vi "Interface.vi"() -> ()   [LabVIEW 2019]
uses:
  <vilib>/Instr/_visa.llb/VISA Configure Serial Port (Instr).vi
  <vilib>/addons/database/Connection.llb/DB Tools Open Connec (Path).vi
  <vilib>/addons/database/Connection.llb/Conn Execute.vi
  <vilib>/addons/database/Recordset.llb/Rec Destroy - Connection.vi
  <vilib>/addons/database/NI_Database_API.lvlib
panel:
  in  "stop":bool
  in  "Pagina":i16(slide) scale=1.0..3.0
  in  "Tab Control":enum32{"INTERFAZ", "ESQUEMA", "INSTRUCCIONES"}(tab)
  in  "VISA resource name":refnum<visa-resource-name>="COM5"
  out "Rt":dbl=100.0 format="%#.2g"
  out "Lectura":dbl
  out "T":dbl=-3.0 format="%#_4g"
  out "Waveform Chart":dbl(graph)=-3.0
  out "Termometro":dbl(slide)=-3.0 scale=10.0..60.0
  # "1.-INTERFAZ\n2.-ESQUEMA\n3.-INSTRUCCIONES"
  # "PÁGINA"
  # "VALORES"
  # "INTERFAZ"
  # "V"
  # "Instrucciones de\nUso en la página 3"
  # "VOLTAJE VAB"
  # "Ohm"
  # "RESISTENCIA PT100"
  # "ºC"
  # "TEMPERATURA"
  # "CIFPN1 Santander"
  # "CONFIGURACIÓN"
  # "(C) 2019"
  # "PUERTO SERIE"
  # "ALBANO DÍEZ DE PAULINO"
  # "ESQUEMA"
  # "Montar como se indica para que funcione correctamente"
  # "Adaptador DB9-USB"
  # "D"
  # "CIFPN1 Santander"
  # "uC ATMEGA328P"
  # "PT100"
  # "C"
  # "5V"
  # "Adaptador TTL-RS232/DB9"
  # "PC"
  # "Puente de Wilson"
  # "D"
  # "C"
  # "INSTRUCCIONES"
  # "Pasos previos antes de ejecutar VI"
  # "INSTRUCCIONES"
  # "1.-Borrar todas las tablas de la base de datos"
  # "1.-Ejecutar VI"
  # "2.-Seleccionar Puerto COM"
  # "2.-No tocar el control del Puerto Serie"
  # "3.-Observar los datos en la grafica y en el termometro"
  # "4.-(Opcional) Parar el programa con el boton STOP"
  # "5.-Esperar a que finalice el programa pasados 5 minutos"
  # "CIFPN1 Santander"
  # "(C) 2019"
  # "ALBANO DÍEZ DE PAULINO"
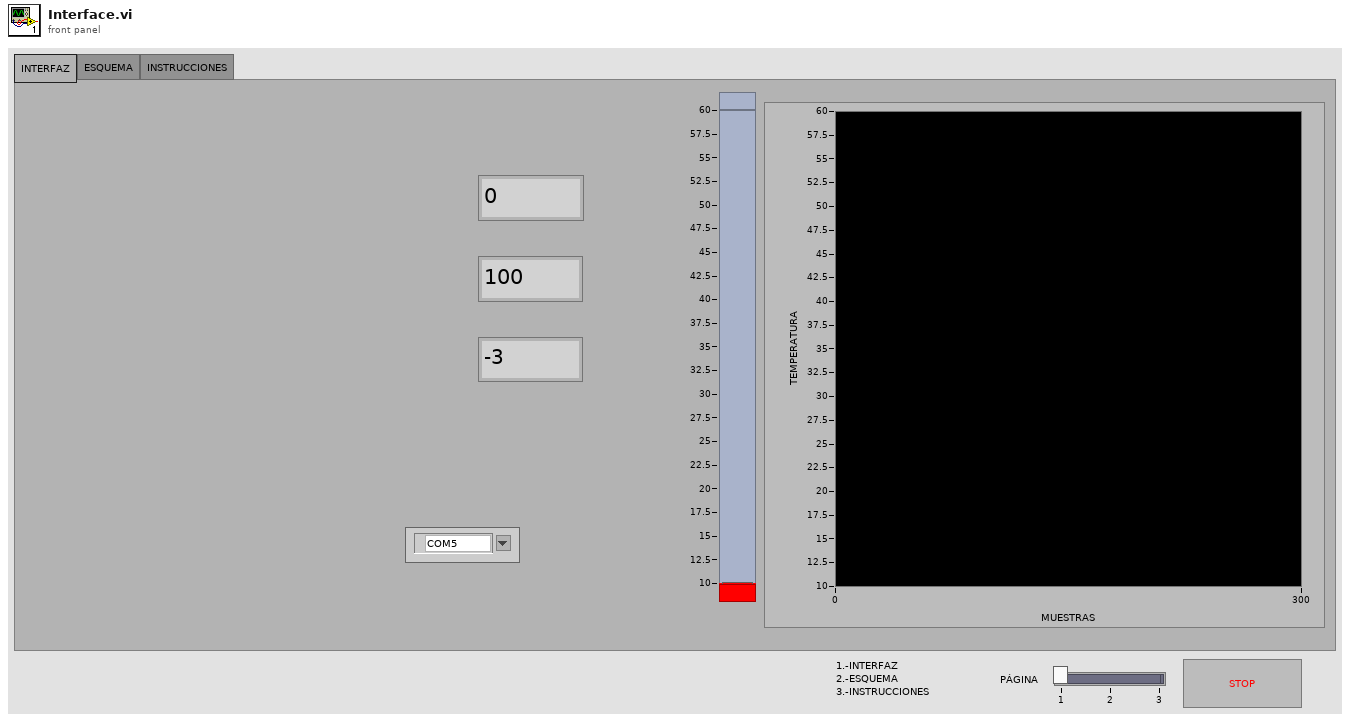
[diagram p1: front panel]
types:
  T1 = enum32{"invalid app kind", "Development System", "Run Time System", "Student Edition", "Embedded LabVIEW", "Evaluation", "Custom"}
  T2 = typedef "NI_Database_API.lvlib/Conn ObjectReference.ctl" = refnum<k1>
  T3 = typedef "NI_Database_API.lvlib/Rec ObjectReference.ctl" = refnum<k1>
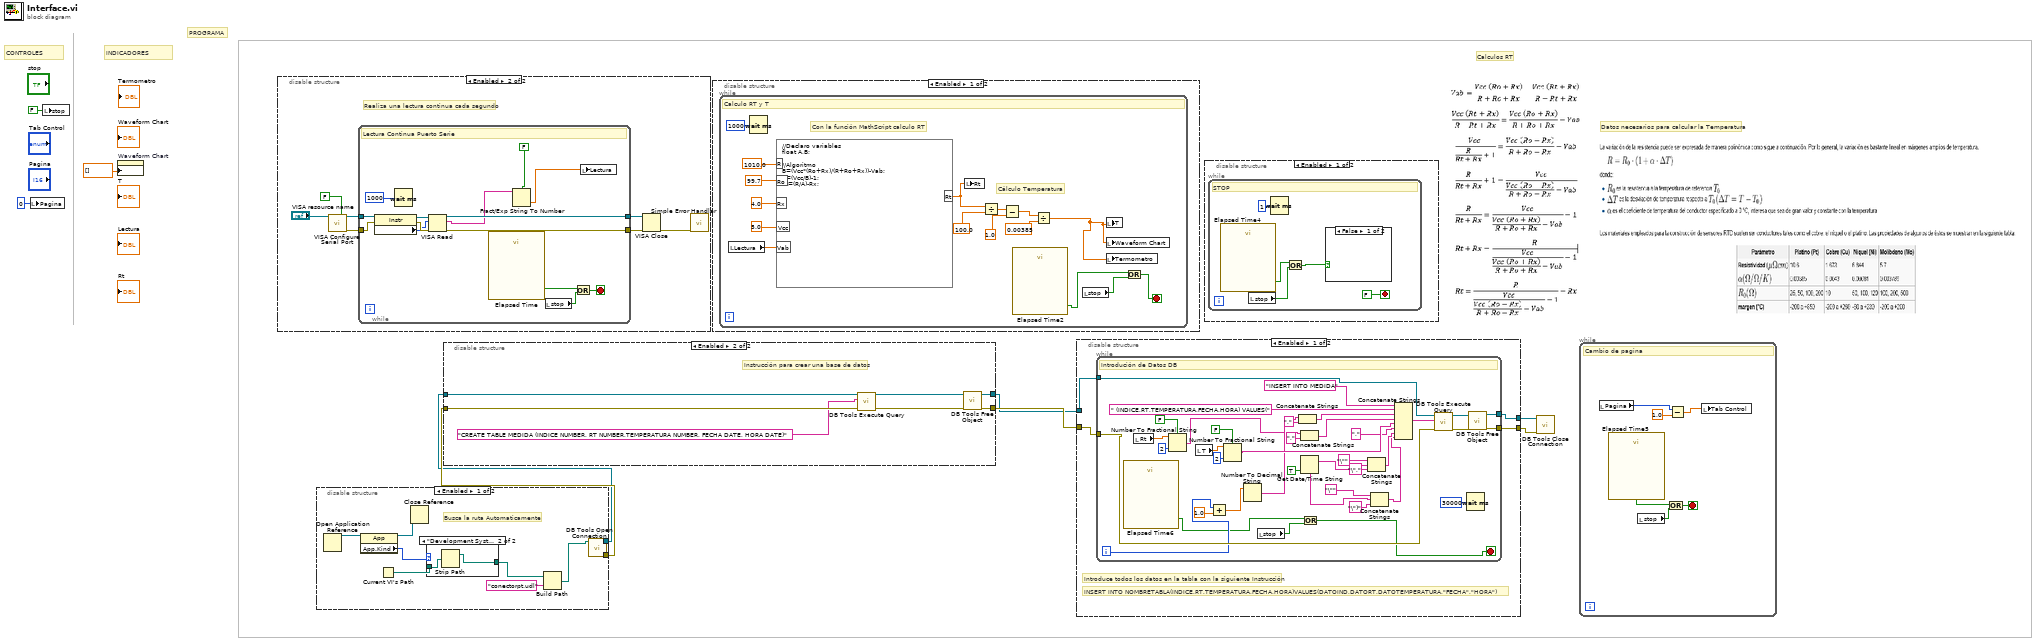
[diagram p0: block diagram]
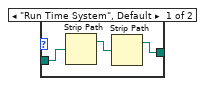
[diagram p3: hidden frame]
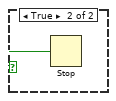
[diagram p6: hidden frame]
diagram:
  # "PROGRAMA"
  # "CONTROLES"
  # "INDICADORES"
  # "Datos necesarios para calcular la Temperatura"
  # "Calculos RT"
  n1 = local write "Pagina"(i16 0 ("Pagina")) -> ()
  n2 = local write "stop"(FALSE ("stop")) -> ()
  n3 = property on="Waveform Chart" class="WFChart (strict)"("History Data"=dbl[] []) -> ()  [unwired: 2 in, 2 out]
  n4 = disable-structure shown="Enabled" {
    frame Disabled {
    }
    frame Enabled {
      # "Realiza una lectura continua cada segundo"
      n5 = call-poly "VISA Configure Serial Port"("VISA resource name"="VISA resource name", "Enable Termination\nChar (T)"=FALSE ("Enable Termination\nChar (T)")) -> ("VISA resource name out"=w14:refnum<visa-resource-name>, "error out"=w15:errorcluster)  [unwired: 8 in, 4 out]
      n6 = while {
        tunnel: w15 -> [w19]
        tunnel: [w28] -> w16
        tunnel: w14 -> [w21]
        tunnel: [w29] -> w13
        stop <- w22 stop-if-true
        # "Lectura Continua Puerto Serie"
        n7 = property class="Instr"(reference=w21, error in=w19) -> (reference out=w20:refnum<visa-resource-name>, error out=w18:errorcluster, "Serial Settings:Number of Bytes at Serial Port"=w17:u32)
        n8 = Wait (ms)(milliseconds to wait=u32 1000) -> ()  [unwired: 1 out]
        n9 = VISA Read(VISA resource name=w20, byte count=w17, error in (no error)=w18) -> (VISA resource name out=w29:refnum<visa-resource-name>, read buffer=w26:string, error out=w28:errorcluster)  [unwired: 1 out]
        n10 = call "Elapsed Time"() -> ("Time has Elapsed"=w23:bool)  [unwired: 12 in, 7 out]
        n11 = Fract/Exp String To Number(use system decimal point (T)=FALSE, string=w26) -> (number=w25:dbl)  [unwired: 2 in, 1 out]
        n12 = local read "stop"() -> (w24:bool)
        n13 = Or(x=w23, y=w24) -> (x .or. y?=w22:bool)
        n14 = local write "Lectura"(w25) -> ()
      }
      n15 = VISA Close(VISA resource name=w13, error in (no error)=w16) -> (error out=w12:errorcluster)
      n16 = call <vilib>:"Simple Error Handler.vi"("error in (no error)"=w12) -> ()  [unwired: 1 in, 8 out]
    }
  }
  n17 = disable-structure shown="Enabled" {
    disable-tunnel: [w39 _] -> w3
    disable-tunnel: [w38 _] -> w4
    frame Enabled {
      # "Busca la ruta Automaticamente"
      n18 = Open Application Reference() -> (3:w37:refnum<vi>)  [unwired: 4 in, 1 out]
      n19 = property class="App"(reference=w37) -> (reference out=w36:refnum<vi>, "App.Kind"=w35:T1)  [unwired: 1 in, 1 out]
      n20 = Current VI's Path() -> (path=w34:path)
      n21 = Close Reference(reference=w36) -> ()  [unwired: 1 in, 1 out]
      n22 = case shown="\"Development System\"" w35 {
        tunnel: w34 -> [w41 w44]
        tunnel: [w40 w43] -> w33
        frame "Run Time System", Default {
          n23 = Strip Path(path=w41) -> (stripped path=w42:path)  [unwired: 1 out]
          n24 = Strip Path(path=w42) -> (stripped path=w40:path)  [unwired: 1 out]
        }
        frame "Development System" {
          n25 = Strip Path(path=w44) -> (stripped path=w43:path)  [unwired: 1 out]
        }
      }
      n26 = Build Path(base path=w33, name or relative path="conectorpt.udl") -> (appended path=w31:path)
      n27 = call-poly <vilib>:"DB Tools Open Connection.vi"("connection information"=w31) -> ("error out"=w38:errorcluster, "connection reference"=w39:T2)  [unwired: 7 in]
    }
    frame Disabled {
    }
  }
  n28 = disable-structure shown="Enabled" {
    disable-tunnel: w3 -> [w45 w53]
    disable-tunnel: w4 -> [w46 w52]
    disable-tunnel: [w46 w51] -> w6
    disable-tunnel: [w45 w50] -> w5
    frame Disabled {
    }
    frame Enabled {
      # "Instrucción para crear una base de datos"
      n29 = call-poly <vilib>:"DB Tools Execute Query.vi"("error in (no error)"=w52, "SQL query"="CREATE TABLE MEDIDA (INDICE NUMBER, RT NUMBER,TEMPERATURA NUMBER, FECHA DATE, HORA DATE)" ("string"), "connection reference"=w53) -> ("error out"=w47:errorcluster, "recordset reference"=w49:T3)  [unwired: 5 in]
      n30 = call-poly <vilib>:"DB Tools Free Object.vi"("error in (no error)"=w47, "recordset reference"=w49) -> ("error out"=w51:errorcluster, "connection reference"=w50:T2)  [unwired: 8 in]
    }
  }
  n31 = disable-structure shown="Enabled" {
    frame Enabled {
      n32 = while {
        stop <- w54 stop-if-true
        # "Cálculo Temperatura"
        # "Con la función MathScript calculo RT"
        # "Calculo RT y T"
        n33 = local read "Lectura"() -> (w64:dbl)
        n34 = Wait (ms)(milliseconds to wait=u32 1000) -> ()  [unwired: 1 out]
        n35 = formula code="//Declaro variables\nfloat A,B;\n\n//Algoritmo\nB=(Vcc*(Ro+Rx)/(R+Ro+Rx))-Vab;\nA=(Vcc/B)-1;\nRt=(R/A)-Rx;"("R"=1010.0 ("input variable"), "Ro"=99.7 ("input variable"), "Rx"=4.0 ("input variable"), "Vcc"=5.0 ("input variable"), "Vab"=w64) -> ("Rt"=w58:dbl)
        n36 = local write "Rt"(w58) -> ()
        n37 = Divide(x=w58, y=100.0) -> (x/y=w62:dbl)
        n38 = Subtract(x=w62, y=1.0) -> (x-y=w60:dbl)
        n39 = call "Elapsed Time2"() -> ("Time has Elapsed"=w55:bool)  [unwired: 12 in, 7 out]
        n40 = Divide(x=w60, y=0.00385) -> (x/y=w57:dbl)
        n41 = local read "stop"() -> (w56:bool)
        n42 = local write "T"(w57) -> ()
        n43 = local write "Waveform Chart"(w57) -> ()
        n44 = local write "Termometro"(w57) -> ()
        n45 = Or(x=w55, y=w56) -> (x .or. y?=w54:bool)
      }
    }
    frame Disabled {
    }
  }
  n46 = disable-structure shown="Enabled" {
    disable-tunnel: w5 -> [w73 _]
    disable-tunnel: w6 -> [w72 _]
    disable-tunnel: [w71 _] -> w2
    disable-tunnel: [w70 _] -> w1
    frame Enabled {
      # "Introduce todos los datos en la tabla con la siguiente Instrucción"
      # "INSERT INTO NOMBRETABLA(INDICE,RT,TEMPERATURA,FECHA,HORA)VALUES(DATOIND,DATORT,DATOTEMPERATURA,\"FECHA\",\"HORA\")"
      n47 = while {
        tunnel: [w108] -> w71
        tunnel: [w107] -> w70
        tunnel: w73 -> [w100]
        tunnel: w72 -> [w99]
        i -> [w85]
        stop <- w74 stop-if-true
        # "Introdución de Datos DB"
        n48 = call "Elapsed Time6"() -> ("Time has Elapsed"=w76:bool)  [unwired: 12 in, 7 out]
        n49 = local read "Rt"() -> (w97:dbl)
        n50 = Number To Fractional String(use system decimal point (T)=FALSE, number=w97, precision (6)=i16 2) -> (F-format string=w80:string)  [unwired: 1 in]
        n51 = local read "T"() -> (w98:dbl)
        n52 = Add(x=w85, y=1.0) -> (x+y=w84:dbl)
        n53 = Number To Fractional String(use system decimal point (T)=FALSE, number=w98, precision (6)=i16 2) -> (F-format string=w92:string)  [unwired: 1 in]
        n54 = Number To Decimal String(number=w84) -> (decimal integer string=w83:string)  [unwired: 1 in]
        n55 = local read "stop"() -> (w77:bool)
        n56 = Concatenate Strings(w83, "," ("string")) -> (w81:string)
        n57 = Concatenate Strings(w80, "," ("string")) -> (w78:string)
        n58 = Get Date/Time String(want seconds? (F)=TRUE) -> (date string=w105:string, time string=w101:string)  [unwired: 2 in]
        n59 = Or(x=w76, y=w77) -> (x .or. y?=w74:bool)
        n60 = Concatenate Strings("\"" ("string"), w105, "\"," ("string")) -> (w90:string)
        n61 = Concatenate Strings("\"" ("string"), w101, "\")" ("string")) -> (w89:string)
        n62 = Concatenate Strings("INSERT INTO MEDIDA" ("string"), " (INDICE,RT,TEMPERATURA,FECHA,HORA) VALUES(" ("string"), w81, w78, w92, "," ("string"), w90, w89) -> (w112:string)
        n63 = call-poly <vilib>:"DB Tools Execute Query.vi"("error in (no error)"=w99, "SQL query"=w112, "connection reference"=w100) -> ("error out"=w111:errorcluster, "recordset reference"=w110:T3)  [unwired: 5 in]
        n64 = Wait (ms)(milliseconds to wait=u32 30000) -> ()  [unwired: 1 out]
        n65 = call-poly <vilib>:"DB Tools Free Object.vi"("error in (no error)"=w111, "recordset reference"=w110) -> ("error out"=w107:errorcluster, "connection reference"=w108:T2)  [unwired: 8 in]
      }
    }
    frame Disabled {
    }
  }
  n66 = disable-structure shown="Enabled" {
    frame Enabled {
      n67 = while {
        stop <- FALSE stop-if-true
        # "STOP"
        n68 = call "Elapsed Time4"() -> ("Time has Elapsed"=w114:bool)  [unwired: 12 in, 7 out]
        n69 = local read "stop"() -> (w115:bool)
        n70 = Wait (ms)(milliseconds to wait=u32 1) -> ()  [unwired: 1 out]
        n71 = Or(x=w114, y=w115) -> (x .or. y?=w113:bool)
        n72 = case shown="False" w113 {
          selector: w113 -> [_ w118]
          frame False {
          }
          frame True {
            n73 = Stop(stop? (T)=w118) -> ()
          }
        }
      }
    }
    frame Disabled {
    }
  }
  n74 = call <vilib>:"DB Tools Close Connection.vi"("error in (no error)"=w1, "connection reference"=w2) -> ()  [unwired: 5 in, 1 out]
  n75 = while {
    stop <- w122 stop-if-true
    # "Cambio de pagina"
    n76 = local read "Pagina"() -> (w119:i16)
    n77 = call "Elapsed Time5"() -> ("Time has Elapsed"=w124:bool)  [unwired: 12 in, 7 out]
    n78 = local read "stop"() -> (w123:bool)
    n79 = Or(x=w124, y=w123) -> (x .or. y?=w122:bool)
    n80 = Subtract(x=w119, y=1.0) -> (x-y=w120:dbl)
    n81 = local write "Tab Control"(w120) -> ()
  }
